vi "Update Strings.vi"(6 "Timestamp (Now)":dbl, 8 "error in (no error)":errorcluster, 10 "Strings":string[](array[string]), 11 "StringGroup in":refnum<class "Group STR.lvclass">) -> (0 "error out":errorcluster, 3 "StringGroup out":refnum<class "Group STR.lvclass">)   [LabVIEW 2020, in "Vecto.lvlib" / "Group STR.lvclass"]
uses:
  Group STR.lvclass
  C:/dev/lv20CE/relink/lv-vecto/Vecto/Group/Group.lvclass
  Group STR.lvclass/Group STR.ctl
  Group/Group.lvclass
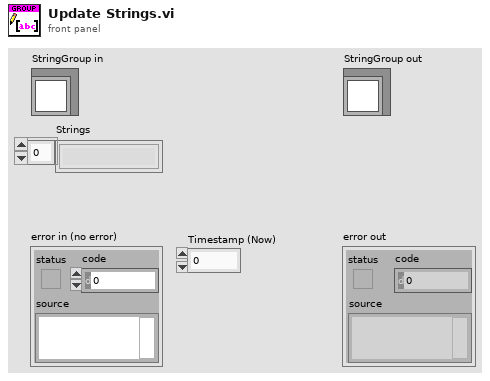
[diagram p1: front panel]
types:
  T1 = typedef "Vecto.lvlib/StringGroup.lvclass/Ref.ctl" = cluster{"Strings":string[], "Timestamp":dbl[]}
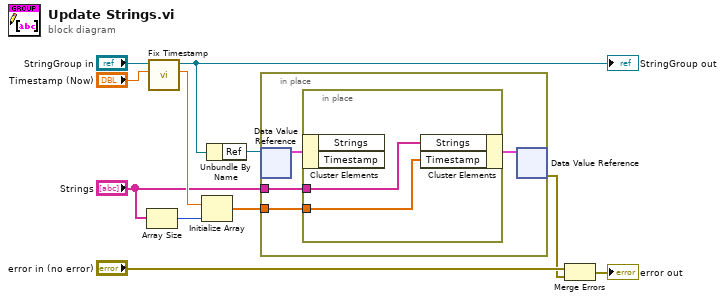
[diagram p0: block diagram]
diagram:
  n1 = Array Size(array="Strings") -> (size(s)=w6:i32)
  n2 = call "Fix Timestamp.vi"("Timestamp in"="Timestamp (Now)", "GroupAbstract in"="StringGroup in") -> ("Timestamp"=w5:dbl, "GroupAbstract out"=w7:refnum<class "Group STR.lvclass">)  [unwired: 7 in, 1 out]
  "StringGroup out" <- w7
  n3 = Initialize Array(w5, w6) -> (w4:dbl[])
  n4 = Unbundle By Name(w7) -> ("Ref"=w8:refnum<data-value>)
  n5 = in-place {
    in-place-border: "Strings" -> [w13]
    in-place-border: w4 -> [w12]
    n6 = in-place-dvr #1(w8) -> (w15:T1)  [unwired: 1 out]
    n7 = in-place {
      in-place-border: w13 -> [w17]
      in-place-border: w12 -> [w16]
      n8 = in-place-cluster #2(w15) -> ()  [unwired: 2 out]
      n9 = in-place-cluster #2("Strings"=w17, "Timestamp"=w16) -> (w14:T1)
    }
    n10 = in-place-dvr #1(w14) -> (w1:errorcluster)  [unwired: 1 out]
  }
  n11 = Merge Errors("error in (no error)", w1) -> (→"error out":errorcluster)
